vi "set_resolution.vi"(8 "error in (no error)":errorcluster, 9 "y":i32, 10 "x":i32, 11 "TrajectoryDL090201FrameScan in":refnum<class "TrajectoryDL090201FrameScan.lvclass">) -> (0 "error out":errorcluster, 3 "TrajectoryDL090201FrameScan out":refnum<class "TrajectoryDL090201FrameScan.lvclass">)   [LabVIEW 2010, in "TrajectoryDL090201FrameScan.lvclass"]
uses:
  TrajectoryDL090201FrameScan.lvclass
  TrajectoryDL090201FrameScan.lvclass/TrajectoryDL090201FrameScan.ctl
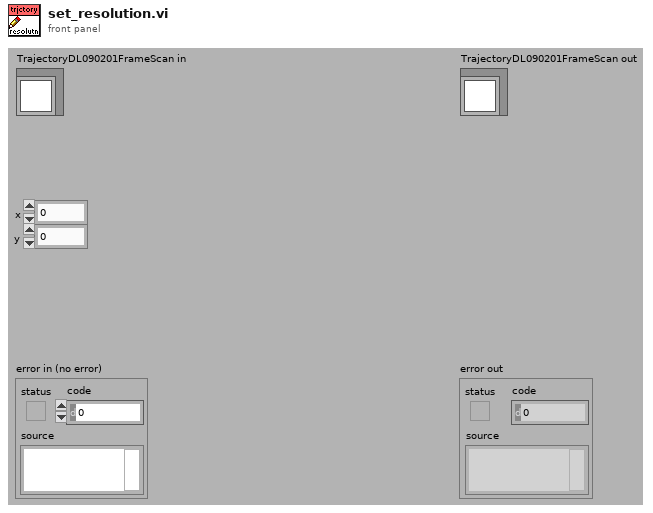
[diagram p1: front panel]
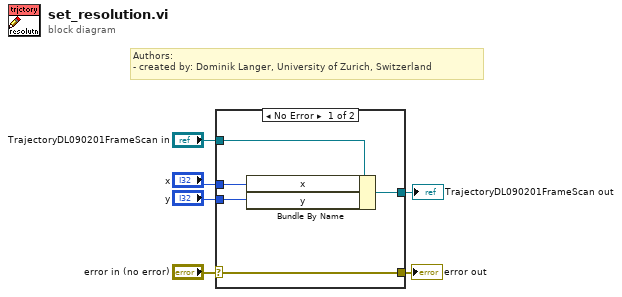
[diagram p0: block diagram]
diagram:
  # "Authors: \n- created by: Dominik Langer, University of Zurich, Switzerland"
  n1 = case shown="No Error" "error in (no error)" {
    selector: "error in (no error)" -> [w11 w12]
    tunnel: [w11 w12] -> w5
    tunnel: [w9 w13] -> w3
    tunnel: "TrajectoryDL090201FrameScan in" -> [w10 w13]
    tunnel: "x" -> [w8 _]
    tunnel: "y" -> [w7 _]
    frame No Error {
      n2 = Bundle By Name(cluster=w10, "x"=w8, "y"=w7) -> (w9:refnum<class "TrajectoryDL090201FrameScan.lvclass">)
    }
    frame Error {
    }
  }
  "error out" <- w5
  "TrajectoryDL090201FrameScan out" <- w3
